vi "Clear Reference Buffer.vi"(8 "error in (no error)":errorcluster, 11 "Ethernet port opened":bool) -> (0 "error out":errorcluster)   [LabVIEW 2020]
panel:
  out "concatenated string":string
  # "This Vi Clears Buffer 1 only \n(Clears Reference Chirp Praameters)"
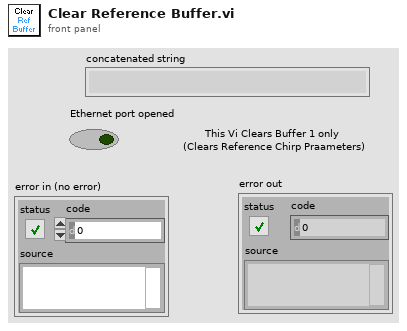
[diagram p1: front panel]
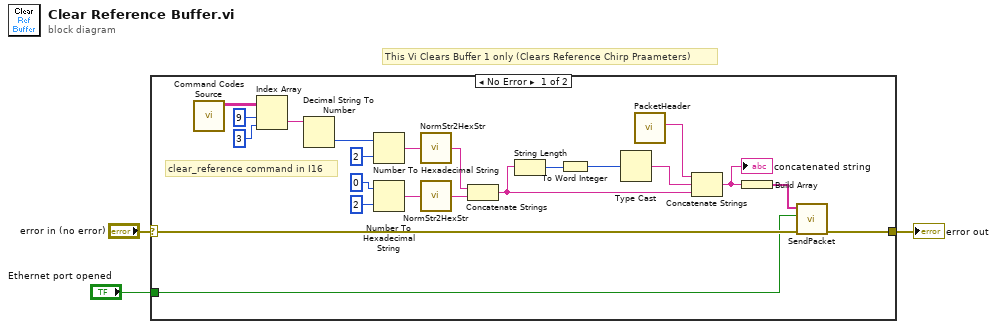
[diagram p0: block diagram]
diagram:
  # "This Vi Clears Buffer 1 only (Clears Reference Chirp Praameters)"
  n1 = case shown="No Error" "error in (no error)" {
    selector: "error in (no error)" -> [w7 w26]
    tunnel: [w8 w26] -> w2
    tunnel: "Ethernet port opened" -> [w4 _]
    frame No Error {
      # "clear_reference command in I16"
      n2 = call "Command Codes Source.vi"() -> ("Commands for FPGA"=w11:string[][])  [unwired: 11 in]
      n3 = Index Array(array=w11, index (row)=9, index (col)=3 ("disabled index (col)")) -> (element=w17:string)
      n4 = Decimal String To Number(string=w17) -> (number=w16:i32)  [unwired: 2 in, 1 out]
      n5 = Number To Hexadecimal String(1:i16 2 ("width (-)"), 2:w16) -> (0:w13:string)
      n6 = Number To Hexadecimal String(1:i16 2 ("width (-)"), 2:u32 0 ("number")) -> (0:w12:string)
      n7 = call "NormStr2HexStr.vi"("string"=w13) -> ("hex string"=w10:string)
      n8 = call "NormStr2HexStr.vi"("string"=w12) -> ("hex string"=w9:string)
      n9 = Concatenate Strings(w10, w9) -> (w25:string)
      n10 = String Length(string=w25) -> (length=w22:i32)
      n11 = To Word Integer(number=w22) -> (16bit integer=w24:i16)
      n12 = Type Cast(x=w24) -> (*(type *) &x=w23:string)  [unwired: 1 in]
      n13 = call "PacketHeader.vi"() -> ("PacketHeader"=w5:string)  [unwired: 11 in]
      n14 = Concatenate Strings(w5, w23, w25) -> (w6:string)
      "concatenated string" <- w6
      n15 = Build Array(w6) -> (w21:string[])
      n16 = call "SendPacket.vi"("error in"=w7, "Ethernet Port Opened ?"=w4, "Packet Array"=w21) -> ("error out"=w8:errorcluster)  [unwired: 7 in, 1 out]
    }
    frame Error {
    }
  }
  "error out" <- w2
